vi "AIT 429 RT Driver VI.vi"(7 "Operation":T1, 11 "Device Reference in":T2 format="%.0x") -> (0 "Error Code":i32)   [LabVIEW 2012, in "AIT 429 Engine.lvlib"]
uses:
  AIT 429 Engine.lvlib
  <vilib>/NI Veristand/Custom Device API/Custom Device Item Ref.ctl
  <vilib>/NI Veristand/Custom Device API/Hardware Interface Driver VI Operation.ctl
  RT Controls/RT Data.ctl
  RT Controls/RT HW Channel.ctl
  RT Controls/RT Label Settings.ctl
  Shared/Controls and Global/Label.ctl
  Shared/Controls and Global/transferPeriod.ctl
  RT Controls/Driver Data.ctl
  RT Controls/RT Word Settings.ctl
  <vilib>/NI Veristand/Custom Device API/Block Data Reference.ctl
  <vilib>/NI Veristand/Custom Device API/Data Reference.ctl
  RT Controls/RT Param Setting.ctl
  Shared/Controls and Global/Start Bit.ctl
  Shared/Controls and Global/Number of Bits.ctl
  Shared/Controls and Global/TransferType.ctl
  RT Controls/Error Qs.ctl
  RT Controls/Status Channels Config.ctl
  RT Controls/FIFO.ctl
  RT Controls/Label Transfer Config.ctl
  RT Controls/Async Loop Control Enum.ctl
  RT Controls/ReadWrite Selector.ctl
  SubVIs/Init/Parse Status Channels.vi
  SubVIs/Init/Get Label Transfer Config Data Refs.vi
  SubVIs/Data Ref FGV.vi
  <vilib>/NI Veristand/Custom Device API/NI VeriStand - Set Channel Value by Data Reference.vi
  SubVIs/Error/Push Error if Different.vi
  SubVIs/ReadWrite/Read FIFOs.vi
  SubVIs/ReadWrite/Write FIFOs.vi
  SubVIs/ReadWrite/ReadWrite TransConfig.vi
  SubVIs/ReadWrite/ReadWrite LoopStats.vi
  SubVIs/Error/Print Error.vi
  <vilib>/NI Veristand/Custom Device API/NI VeriStand - Get Channel Values by Block Data Reference.vi
  SubVIs/Init/Parse Channels.vi
  Shared/Controls and Global/Global.vi
  <vilib>/NI Veristand/Custom Device API/NI VeriStand - Get Channel Data Reference.vi
  <vilib>/NI Veristand/Custom Device Tools/Custom Device Utility Library/NI VeriStand - Search for Item.vi
  <vilib>/NI Veristand/Custom Device Tools/Custom Device Utility Library/NI VeriStand - Search for Item by Name.vi
  <vilib>/NI Veristand/Custom Device API/NI VeriStand - Get Item Reference by Name.vi
  <vilib>/NI Veristand/Custom Device API/NI VeriStand - Get Channel Block Data References.vi
  <vilib>/NI Veristand/Custom Device Tools/Custom Device Utility Library/NI VeriStand - Search for All Items by GUID.vi
  <vilib>/NI Veristand/Custom Device Tools/Custom Device Utility Library/NI VeriStand - Search for Item by GUID.vi
  <vilib>/NI Veristand/Custom Device API/Global Data Refs.vi
  SubVIs/ReadWrite/ReadWrite All Data.vi
  <instrlib>/AIT 429/AIT 429.lvlib
  Shared/ARINC 429 Shared.lvlib
  <vilib>/NI Veristand/Custom Device API/Custom Device API.lvlib
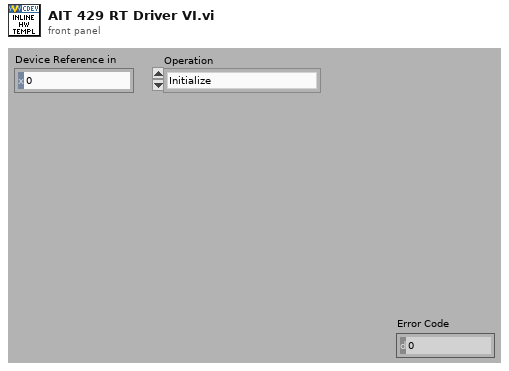
[diagram p1: front panel]
types:
  T1 = typedef "Custom Device API.lvlib/Hardware Interface Driver VI Operation.ctl" = enum16{"Initialize", "Start", "Read Data from HW", "Write Data to HW", "Close"}
  T2 = typedef "Custom Device API.lvlib/Custom Device Item Ref.ctl" = u64
  T3 = typedef "AIT 429 Engine.lvlib/RT Data.ctl" = cluster{"HWInput Channels":T4[], "HWOutput Channels":T4[], "board handle":u32, "Start":refnum<notifier>, "HWIn BaseRate":i64, "HWOut BaseRate":i64, "Error Qs":T16, "Error Pub Q":refnum<queue>, "Status Config":T17, "FIFOs":T18, "VI Refs":refnum<vi>[], "Label Transfer Config":T19, "ScheduledSDI":bool}
  T4 = typedef "AIT 429 Engine.lvlib/RT HW Channel.ctl" = cluster{"Labels Settings":T5[], "channel handle":u32, "channel #":u16, "Label Map":i32[], "Label Buffer":u32[], "rdBufHandle":u32}
  T5 = typedef "AIT 429 Engine.lvlib/RT Label Settings.ctl" = cluster{"Name":string, "xmlName":string, "Label":T6, "transferPeriod":T7, "Driver Data":T8, "SDI_Enabled":bool, "SDI":u8, "Words":T9[], "bufferSize":u32, "RxWordIdx":i32, "TxWordIdx":i32, "TransferType":T15, "has timestamp?":bool}
  T6 = typedef "ARINC 429 Shared.lvlib/Label.ctl" = u8
  T7 = typedef "ARINC 429 Shared.lvlib/transferPeriod.ctl" = u32
  T8 = typedef "AIT 429 Engine.lvlib/Driver Data.ctl" = cluster{"Lbl Tx Hdl":u32, "Decimation":i32, "IterationOffset":i32, "transfer handle":u32, "RX Word":u32, "TXChange":bool, "RX timestamp":dbl}
  T9 = typedef "AIT 429 Engine.lvlib/RT Word Settings.ctl" = cluster{"Block Data Refs":T10[], "Values Array":dbl[], "Length":i32, "FIFO Index":i32, "Param Setting":T12}
  T10 = typedef "Custom Device API.lvlib/Block Data Reference.ctl" = cluster{"Data Reference":T11, "Offset":i32, "Length":i32}
  T11 = typedef "Custom Device API.lvlib/Data Reference.ctl" = i32
  T12 = typedef "AIT 429 Engine.lvlib/RT Param Setting.ctl" = cluster{"Start Bit":T13[], "Num Bits":T14[], "Signed?":bool[], "ScaleFac":dbl[], "ScaleOffset":dbl[]}
  T13 = typedef "ARINC 429 Shared.lvlib/Start Bit.ctl" = i32
  T14 = typedef "ARINC 429 Shared.lvlib/Number of Bits.ctl" = i32
  T15 = typedef "ARINC 429 Shared.lvlib/TransferType.ctl" = enum16{"ScheduledLabel", "Acyclic", "Block", "Strobe"}
  T16 = typedef "AIT 429 Engine.lvlib/Error Qs.ctl" = cluster{"HWIn":refnum<queue>, "HWOut":refnum<queue>, "TransCfg":refnum<queue>}
  T17 = typedef "AIT 429 Engine.lvlib/Status Channels Config.ctl" = cluster{"Error Data Ref":T11, "HWIn Dur Ref":T11, "HWIn Dur Idx":i32, "HWOut Dur Ref":T11, "HWOut Dur Idx":i32}
  T18 = typedef "AIT 429 Engine.lvlib/FIFO.ctl" = cluster{"From HWIn":refnum<k33>, "To HWOut":refnum<k33>, "From HWIn Buf":dbl[], "To HWOut Buf":dbl[], "To TansCfg":refnum<k33>, "To TransCfg Buf":dbl[], "From HWOut":refnum<k33>, "From HWOut Buf":dbl[], "Old To HWOut Buf":dbl[]}
  T19 = typedef "AIT 429 Engine.lvlib/Label Transfer Config.ctl" = cluster{"Block Data Refs":T10[], "Values Array":dbl[]}
  T20 = typedef "AIT 429 Engine.lvlib/Async Loop Control Enum.ctl" = enum16{"Launch", "Start", "Stop"}
  T21 = typedef "AIT 429 Engine.lvlib/ReadWrite Selector.ctl" = enum16{"Inline Read", "Inline Write", "Async HWIn", "Async HWOut"}
  T22 = typedef "AIT 429 Engine.lvlib/FIFO Idx Qs.ctl" = cluster{"From HWInput":refnum<queue>, "To HWOutput":refnum<queue>, "From HWOutput":refnum<queue>}
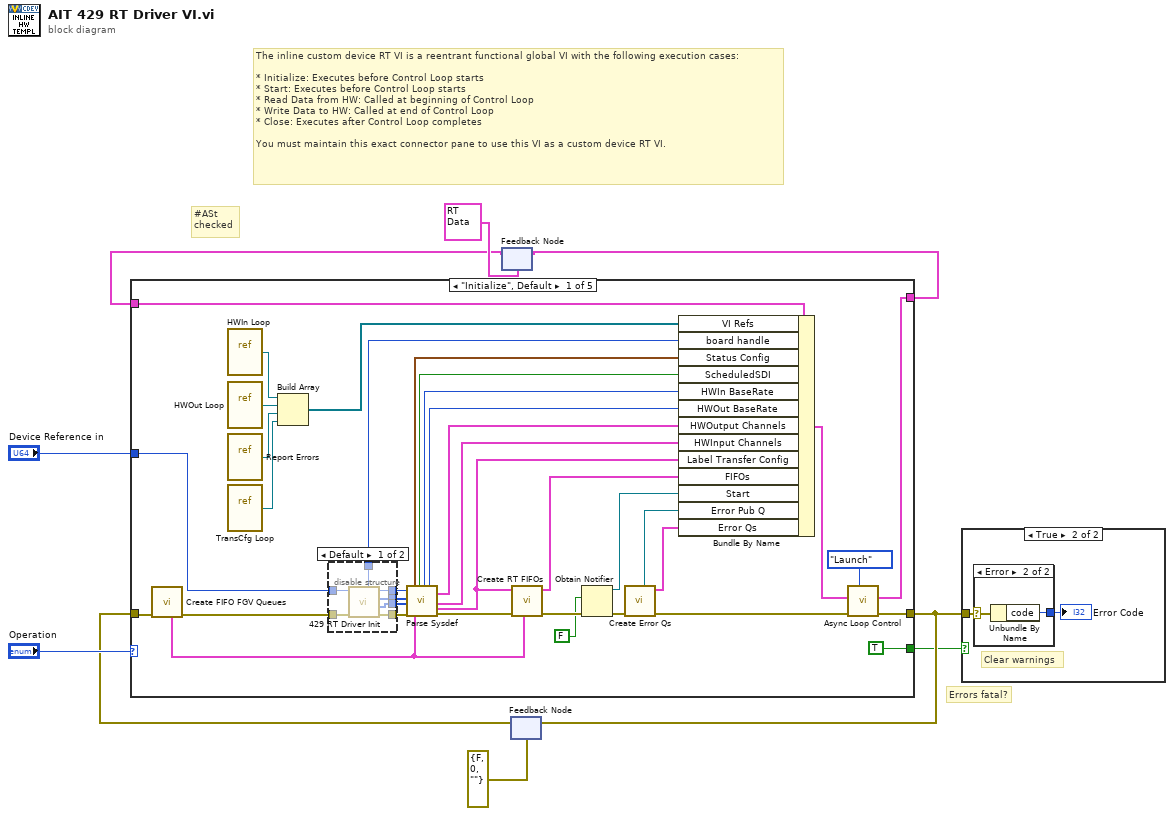
[diagram p0: block diagram]
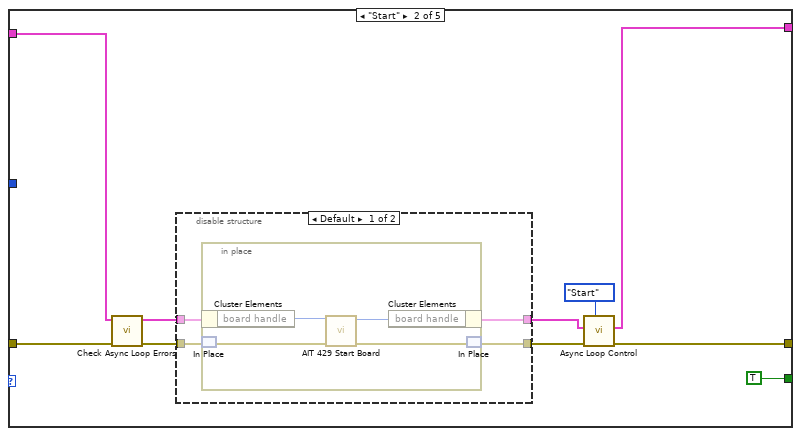
[diagram p5: hidden frame]
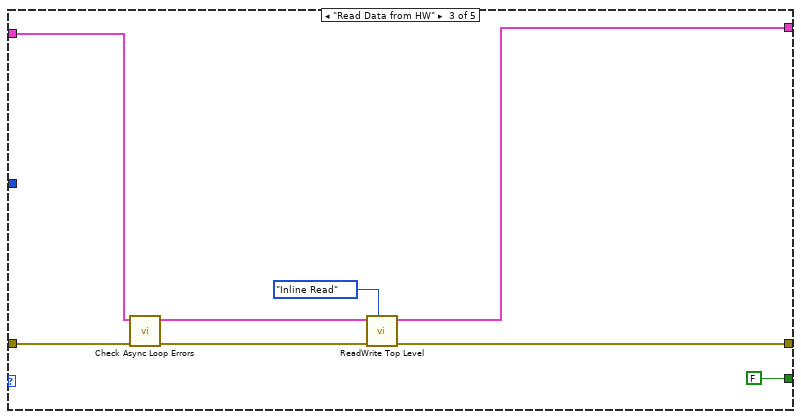
[diagram p7: hidden frame]
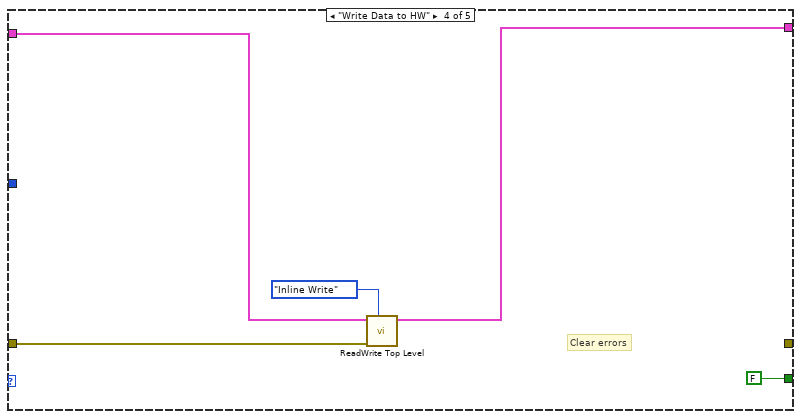
[diagram p8: hidden frame]
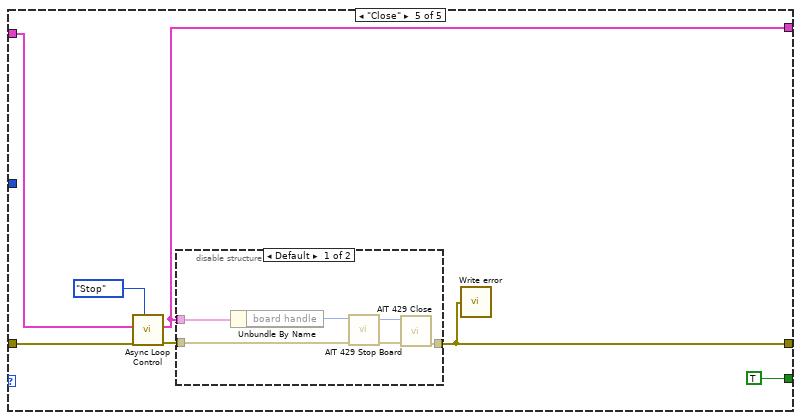
[diagram p9: hidden frame]
diagram:
  # "#ASt\nchecked"
  # "Errors fatal?"
  # "The inline custom device RT VI is a reentrant functional global VI with the following execution cases:\n\n* Initialize: Executes before Control Loop starts\n* Start: Executes before Control Loop starts\n* Read Data from HW: Called at beginning of Control Loop\n* Write Data to HW: Called at end of Control Loop\n* Close: Executes after Control Loop completes\n\nYou must maintain this exact connector pane to use this VI as a custom device RT VI."
  n1 = feedback #1(T3 {"HWInput Channels"=[], "HWOutput Channels"=[], "board handle"=0, "Start"=refnum, "HWIn BaseRate"=0, "HWOut BaseRate"=0, "Error Qs"={"HWIn"=refnum, "HWOut"=refnum, "TransCfg"=refnum}, "Error Pub Q"=refnum, "Status Config"={"Error Data Ref"=0, "HWIn Dur Ref"=0, "HWIn Dur Idx"=0, "HWOut Dur Ref"=0, "HWOut Dur Idx"=0}, "FIFOs"={"From HWIn"=refnum, "To HWOut"=refnum, "From HWIn Buf"=[], "To HWOut Buf"=[], "To TansCfg"=refnum, "To TransCfg Buf"=[], "From HWOut"=refnum, "From HWOut Buf"=[], "Old To HWOut Buf"=[]}, "VI Refs"=[], "Label Transfer Config"={"Block Data Refs"=[], "Values Array"=[]}, "ScheduledSDI"=FALSE} ("RT Data")) -> (w2:T3)
  n2 = feedback #2(errorcluster {"status"=FALSE, "code"=0, "source"=""} ("error out")) -> (w6:errorcluster)
  n3 = case shown="\"Initialize\", Default" "Operation" {
    tunnel: w2 -> [w24 w62 w79 w87 w89]
    tunnel: "Device Reference in" -> [w28 _ _ _ _]
    tunnel: [w37 w55 w81 w86 w88] -> w1
    tunnel: [w42 w63 w82 _ w92] -> w7
    tunnel: w6 -> [w36 w61 w76 w84 w91]
    tunnel: [TRUE TRUE FALSE FALSE TRUE] -> w5
    frame "Initialize", Default {
      n4 = call "Create FIFO FGV Queues.vi"("error in (no error)"=w36) -> ("error out"=w30:errorcluster, "FIFO Idx Qs"=w35:T22)  [unwired: 9 in]
      n5 = vi-ref "HWIn Loop.vi"() -> (w32:refnum<vi>)
      n6 = vi-ref "HWOut Loop.vi"() -> (w33:refnum<vi>)
      n7 = vi-ref "Report Errors.vi"() -> (w34:refnum<vi>)
      n8 = vi-ref "TransCfg Loop.vi"() -> (w31:refnum<vi>)
      n9 = Build Array(w32, w33, w34, w31) -> (w13:refnum<vi>[])
      n10 = disable-structure shown="Default" {
        disable-tunnel: w30 -> [w52 w53]
        disable-tunnel: [w51 w53] -> w29
        disable-tunnel: w28 -> [w50 w54]
        disable-tunnel: [w49 w54] -> w27
        disable-tunnel: [w48 _] -> w26
        disable-tunnel: [w47 _] -> w25
        disable-tunnel: [w46 _] -> w12
        frame condition #0 {
          n11 = call "429 RT Driver Init.vi"("error in"=w52, "Device Reference in"=w50) -> ("error out"=w51:errorcluster, "tx channel handle array"=w47:u32[], "rx channel handle array"=w48:u32[], "Device Reference out"=w49:T2, "board handle"=w46:u32)  [unwired: 5 in]
        }
        frame condition #1 (active) {
        }
      }
      n12 = call "Parse Sysdef.vi"("Device Reference in"=w27, "rx channel handle array"=w26, "tx channel handle array"=w25, "error in (no error)"=w29, "FIFO Idx Qs"=w35) -> ("Status Config"=w11:T17, "ScheduledSDI"=w10:bool, "HWIn BaseRate"=w14:i32, "HWOut BaseRate"=w15:i32, "HWOutput Section Data"=w16:T4[], "HWInput Section Data"=w17:T4[], "Label Transfer Config"=w18:T19, "error out"=w45:errorcluster)  [unwired: 6 in, 1 out]
      n13 = call "Create RT FIFOs.vi"("FIFO Idx Qs"=w35, "error in (no error)"=w45, "Label Transfer Config"=w18) -> ("error out"=w44:errorcluster, "output cluster"=w19:T18)  [unwired: 7 in]
      n14 = Obtain Notifier(notification data type=FALSE, error in (no error)=w44) -> (notifier out=w20:refnum<notifier>, error out=w40:errorcluster)  [unwired: 2 in, 1 out]
      n15 = call "Create Error Qs.vi"("error in (no error)"=w40) -> ("error out"=w39:errorcluster, "Error Qs"=w22:T16, "Error Publishing Q"=w21:refnum<queue>)  [unwired: 8 in]
      n16 = Bundle By Name(cluster=w24, "VI Refs"=w13, "board handle"=w12, "Status Config"=w11, "ScheduledSDI"=w10, "HWIn BaseRate"=w14, "HWOut BaseRate"=w15, "HWOutput Channels"=w16, "HWInput Channels"=w17, "Label Transfer Config"=w18, "FIFOs"=w19, "Start"=w20, "Error Pub Q"=w21, "Error Qs"=w22) -> (w23:T3)
      n17 = call "Async Loop Control.vi"("Action"=Async_Loop_Control_Enum."Launch", "error in (no error)"=w39, "RT Data In"=w23) -> ("error out"=w42:errorcluster, "RT Data Out"=w37:T3)  [unwired: 7 in]
    }
    frame "Start" {
      n18 = call "Check Async Loop Errors.vi"("error in (no error)"=w61, "RT Data in"=w62) -> ("error out"=w59:errorcluster, "RT Data Out"=w58:T3)  [unwired: 8 in]
      n19 = disable-structure shown="Default" {
        disable-tunnel: w59 -> [w68 w73]
        disable-tunnel: w58 -> [w67 w74]
        disable-tunnel: [w66 w74] -> w57
        disable-tunnel: [w65 w73] -> w56
        frame condition #0 {
          n20 = in-place {
            n21 = in-place-cluster #3(w67) -> ("board handle"=w70:u32)
            n22 = in-place-match #4(w68) -> (w72:errorcluster)
            n23 = call <instrlib>:"AIT 429 Start Board.vi"("error in (no error)"=w72, "board handle"=w70) -> ("error out"=w71:errorcluster, "board handle"=w69:u32)  [unwired: 8 in]
            n24 = in-place-cluster #3("board handle"=w69) -> (w66:T3)
            n25 = in-place-match #4(w71) -> (w65:errorcluster)
          }
        }
        frame condition #1 (active) {
        }
      }
      n26 = call "Async Loop Control.vi"("Action"=Async_Loop_Control_Enum."Start", "error in (no error)"=w56, "RT Data In"=w57) -> ("error out"=w63:errorcluster, "RT Data Out"=w55:T3)  [unwired: 7 in]
    }
    frame "Read Data from HW" {
      n27 = call "Check Async Loop Errors.vi"("error in (no error)"=w76, "RT Data in"=w79) -> ("error out"=w77:errorcluster, "RT Data Out"=w78:T3)  [unwired: 8 in]
      n28 = call "ReadWrite Top Level.vi"("Mode"=ReadWrite_Selector."Inline Read", "error in (no error)"=w77, "RT Data in"=w78) -> ("error out"=w82:errorcluster, "RT Data out"=w81:T3)  [unwired: 7 in]
    }
    frame "Write Data to HW" {
      # "Clear errors"
      n29 = call "ReadWrite Top Level.vi"("Mode"=ReadWrite_Selector."Inline Write", "error in (no error)"=w84, "RT Data in"=w87) -> ("RT Data out"=w86:T3)  [unwired: 7 in, 1 out]
    }
    frame "Close" {
      n30 = call "Async Loop Control.vi"("Action"=Async_Loop_Control_Enum."Stop", "error in (no error)"=w91, "RT Data In"=w89) -> ("error out"=w94:errorcluster, "RT Data Out"=w88:T3)  [unwired: 7 in]
      n31 = disable-structure shown="Default" {
        disable-tunnel: w94 -> [w99 w101]
        disable-tunnel: [w98 w101] -> w92
        disable-tunnel: w88 -> [w95 _]
        frame condition #0 {
          n32 = Unbundle By Name(w95) -> ("board handle"=w100:u32)
          n33 = call <instrlib>:"AIT 429 Stop Board.vi"("error in (no error)"=w99, "board handle"=w100) -> ("error out"=w97:errorcluster, "board handle"=w96:u32)  [unwired: 8 in]
          n34 = call <instrlib>:"AIT 429 Close.vi"("error in (no error)"=w97, "board handle"=w96) -> ("error out"=w98:errorcluster)  [unwired: 9 in]
        }
        frame condition #1 (active) {
        }
      }
      n35 = call "Write error.vi"("error in (no error)"=w92) -> ()
    }
  }
  n36 = feedback-in #1(w1) -> ()
  n37 = feedback-in #2(w7) -> ()
  n38 = case shown="True" w5 {
    tunnel: w7 -> [_ w102]
    frame False {
    }
    frame True {
      # "Clear warnings"
      n39 = case shown="Error" w102 {
        selector: w102 -> [_ w105]
        tunnel: [_ w104] -> w103
        frame No Error {
        }
        frame Error {
          n40 = Unbundle By Name(w105) -> ("code"=w104:i32)
        }
      }
      "Error Code" <- w103
    }
  }
